vi "Query Platform Instrument Catalog Full.vi"(8 "error in (no error)":errorcluster, 10 "Query Catalog (0:Instrument Catalog)":u16(ring) items=["Instrument Catalog", "Instrument Catalog Full"], 11 "VISA resource name":refnum<visa-resource-name>) -> (0 "error out":errorcluster, 2 "Catalog Full":string, 3 "VISA resource name out":refnum<visa-resource-name>)   [LabVIEW 2018, in "LTB-1.lvlib" / "3150.lvlib"]
doc: "Queries the instrument catalog from two commands. The commands return list of string - integer pairs. The string contains the name of the logical instrument. The immediately following integer formatted number is its associated logical instrument number. All response data elements are separated by commas. If no logical instrument is defined, a null string value followed by a zero is returned."
uses:
  3150.lvlib
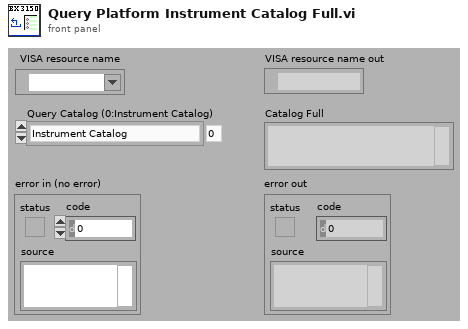
[diagram p1: front panel]
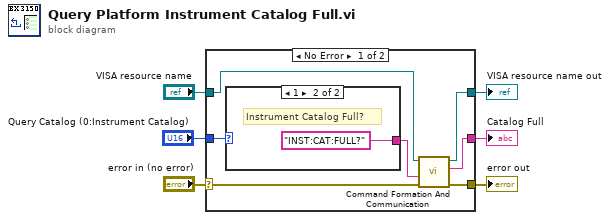
[diagram p0: block diagram]
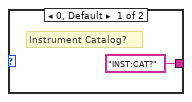
[diagram p2: hidden frame]
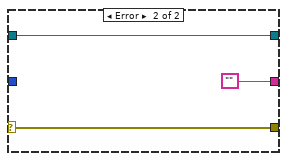
[diagram p3: hidden frame]
diagram:
  n1 = case shown="No Error" "error in (no error)" {
    selector: "error in (no error)" -> [w13 w18]
    tunnel: [w10 w17] -> w6
    tunnel: [w12 w18] -> w3
    tunnel: [w11 ""] -> w2
    tunnel: "VISA resource name" -> [w9 w17]
    tunnel: "Query Catalog (0:Instrument Catalog)" -> [w8 _]
    frame No Error {
      n2 = case shown="1" w8 {
        tunnel: ["INST:CAT?" ("Command") "INST:CAT:FULL?" ("Command")] -> w7
        frame 0, Default {
          # "Instrument Catalog?"
        }
        frame 1 {
          # "Instrument Catalog Full?"
        }
      }
      n3 = call "Command Formation And Communication.vi"("error in (no error)"=w13, "Command"=w7, "VISA resource name"=w9) -> ("error out"=w12:errorcluster, "Response"=w11:string, "VISA resource name out"=w10:refnum<visa-resource-name>)  [unwired: 1 in, 5 out]
    }
    frame Error {
    }
  }
  "VISA resource name out" <- w6
  "error out" <- w3
  "Catalog Full" <- w2
